vi "Flip Mirror Manual.vi"(8 "error in (no error)":errorcluster, 11 "Manual Mirror":T1) -> (0 "error out":errorcluster, 3 "Mirrors":T2)   [LabVIEW 2016]
uses:
  Controls/Flip Mirrors.ctl
  Controls/Mirror Data.ctl
  Controls/Flip Mirror Manual.ctl
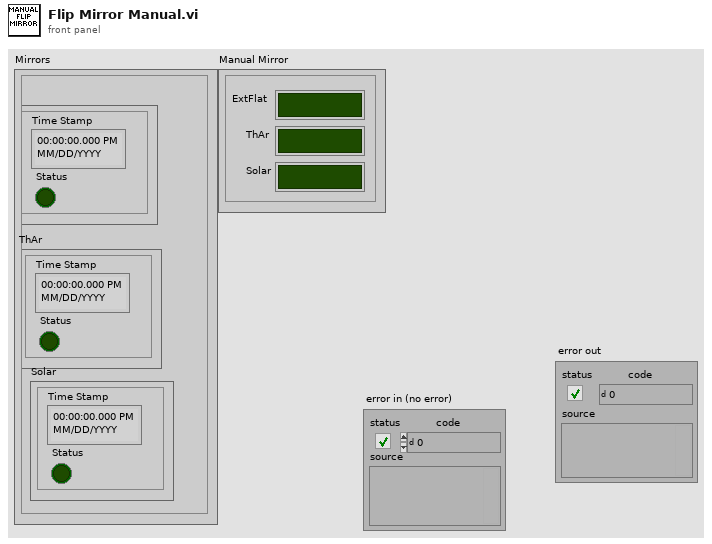
[diagram p1: front panel]
types:
  T1 = typedef "Flip Mirror Manual.ctl" = cluster{"ExtFlat":bool, "Solar":bool, "ThAr":bool}
  T2 = typedef "Flip Mirrors.ctl" = cluster{"ExtFlat":T3, "ThAr":T3, "Solar":T3}
  T3 = typedef "Mirror Data.ctl" = cluster{"Status":bool, "Time Stamp":timestamp}
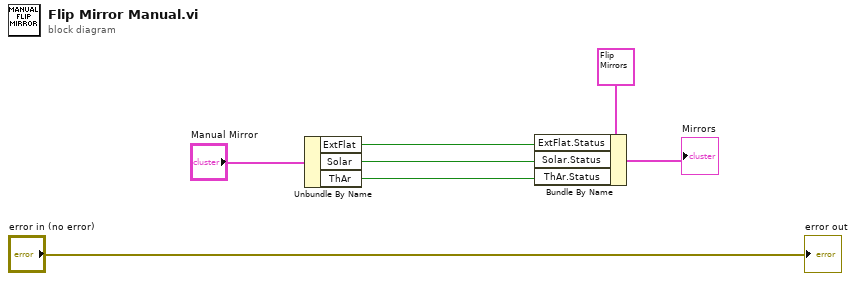
[diagram p0: block diagram]
diagram:
  n1 = Unbundle By Name("Manual Mirror") -> ("ExtFlat"=w4:bool, "Solar"=w3:bool, "ThAr"=w2:bool)
  n2 = Bundle By Name(cluster=T2 {"ExtFlat"={"Status"=FALSE, "Time Stamp"=timestamp(0 s since 1904-01-01)}, "ThAr"={"Status"=FALSE, "Time Stamp"=timestamp(0 s since 1904-01-01)}, "Solar"={"Status"=FALSE, "Time Stamp"=timestamp(0 s since 1904-01-01)}} ("Mirrors 2"), "ExtFlat.Status"=w4, "Solar.Status"=w3, "ThAr.Status"=w2) -> (→"Mirrors":T2)
  "error out" <- "error in (no error)"
